vi "Read_Parameters_From_Data_Packet.vi"(8 "error in (no error)":errorcluster, 11 "Data_Packet in":T1={"Packet"={"Raw Bytes"=[], "Checksum"=FALSE, "Direction"=enum."Transmit", "Processed Bytes"=[], "Node ID"=0, "Packet type"=enum."Connection Management", "Frame Data"=0, "Priority"=enum."LOW", "Frame ID"=0}, "Parameters"=[], "Last Received Time (ms)"=0, "Receive count"=0, "Transmit count"=0, "Transmit interval (ms)"=0, "Last Transmitted Time (ms)"=0, "Receive interval (ms)"=0, "Transmit_Mode"=enum."Disabled", "Transmit Enable"=FALSE, "Cyclic Transmit interval (ms)"=0}) -> (0 "error out":errorcluster, 2 "Data Packets Out":T1[](array[typedef]), 3 "Data_Packet out":T1={"Packet"={"Raw Bytes"=[], "Checksum"=FALSE, "Direction"=enum."Transmit", "Processed Bytes"=[], "Node ID"=0, "Packet type"=enum."Connection Management", "Frame Data"=0, "Priority"=enum."LOW", "Frame ID"=0}, "Parameters"=[], "Last Received Time (ms)"=0, "Receive count"=0, "Transmit count"=0, "Transmit interval (ms)"=0, "Last Transmitted Time (ms)"=0, "Receive interval (ms)"=0, "Transmit_Mode"=enum."Disabled", "Transmit Enable"=FALSE, "Cyclic Transmit interval (ms)"=0})   [LabVIEW 2017]
uses:
  Controls/Data Packets/Data_Packet.ctl
  Controls/Packet/Packet.ctl
  Controls/Packet/Packet_Direction.ctl
  Controls/Packet/Packet_Type.ctl
  Controls/Packet/Packet_Priority.ctl
  Controls/Data Packets/Parameter.ctl
  Controls/Data Packets/Parameter_Data_Type.ctl
  Controls/Data Packets/Data_Packet_Transmit_Mode.ctl
  Controls/Data Packets/Data_Packet_FGV_Commands.ctl
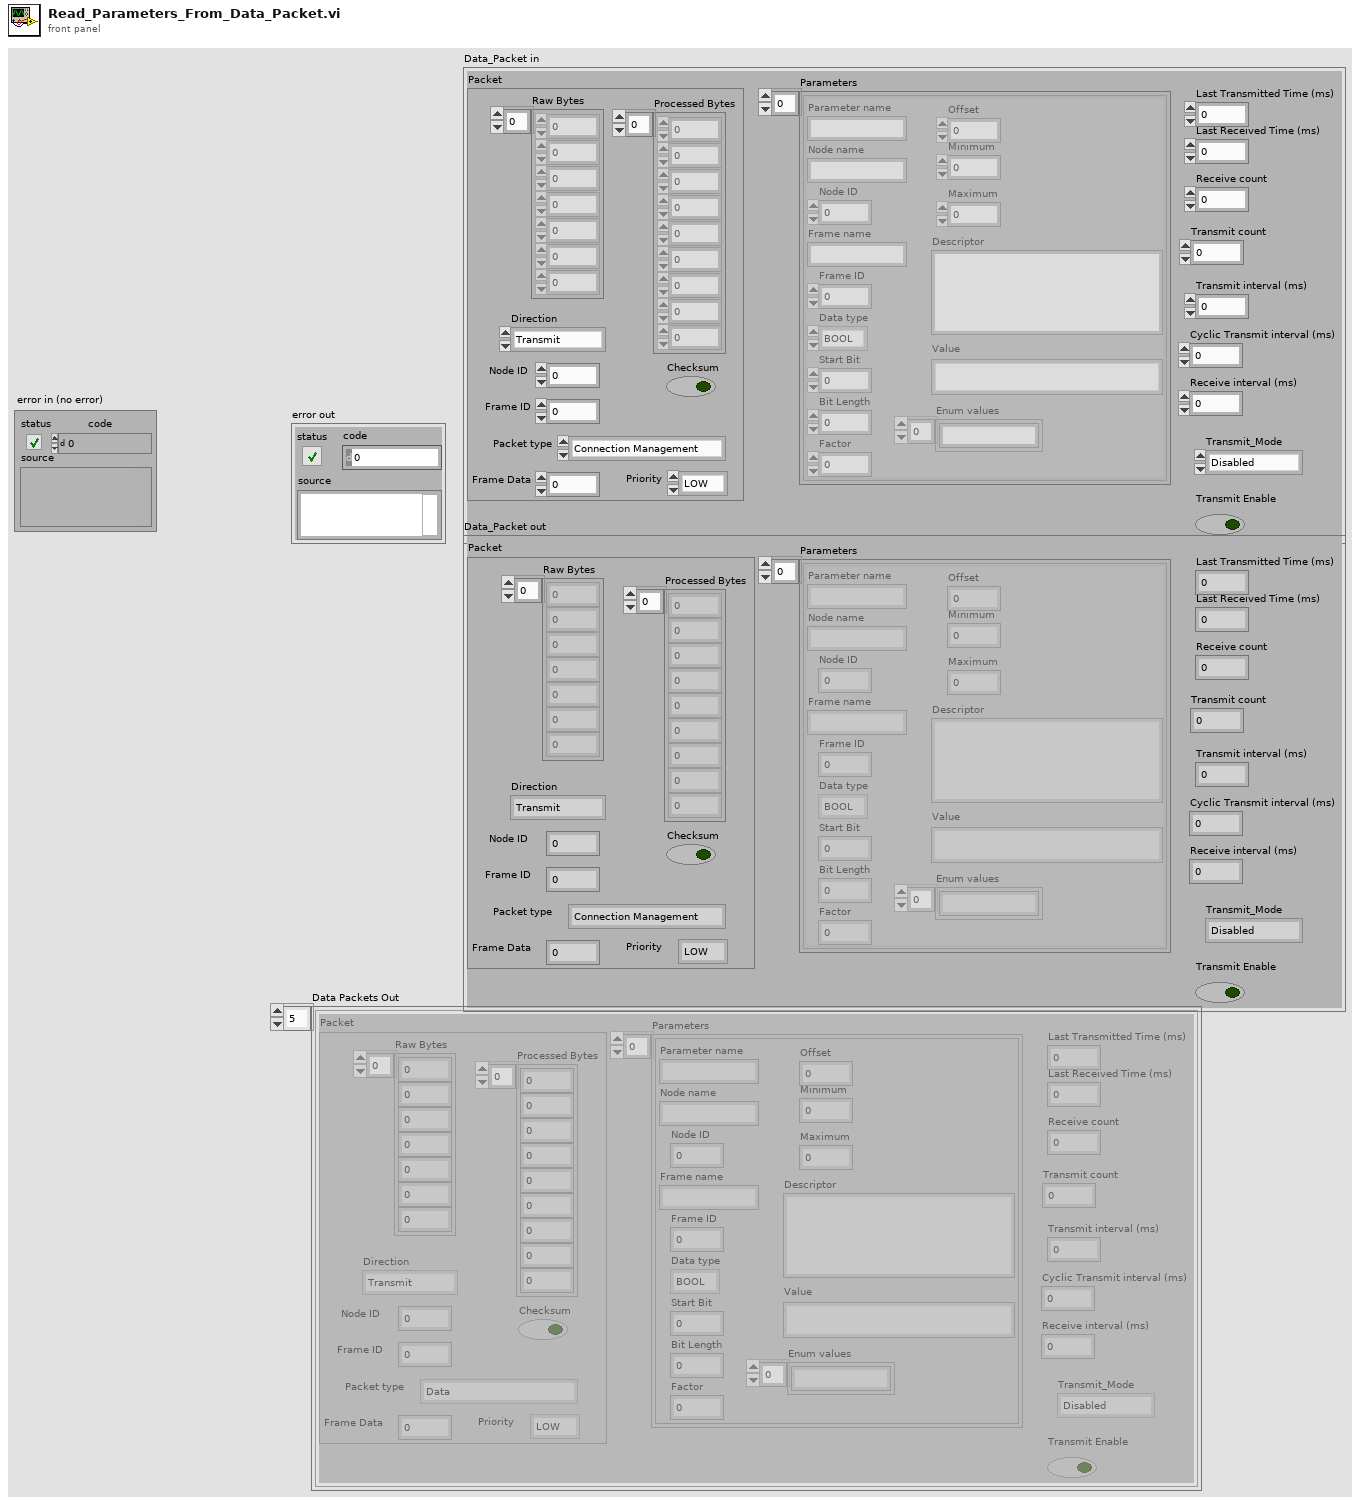
[diagram p1: front panel]
types:
  T1 = typedef "Data_Packet.ctl" = cluster{"Packet":T2, "Parameters":T6[], "Last Received Time (ms)":u64, "Receive count":i32, "Transmit count":i32, "Transmit interval (ms)":u32, "Last Transmitted Time (ms)":u64, "Receive interval (ms)":u32, "Transmit_Mode":T8, "Transmit Enable":bool, "Cyclic Transmit interval (ms)":u32}
  T2 = typedef "Packet.ctl" = cluster{"Raw Bytes":u8[], "Checksum":bool, "Direction":T3, "Processed Bytes":u8[], "Node ID":u8, "Packet type":T4, "Frame Data":u32, "Priority":T5, "Frame ID":u8}
  T3 = typedef "Packet_Direction.ctl" = enum16{"Transmit", "Receive", "Bidirectional"}
  T4 = typedef "Packet_Type.ctl" = enum16{"Data", "Connection Management", "Remote Request", "Error/Status"}
  T5 = typedef "Packet_Priority.ctl" = enum16{"LOW", "HIGH"}
  T6 = typedef "Parameter.ctl" = cluster{"Parameter name":string, "Node name":string, "Node ID":u8, "Frame name":string, "Frame ID":u8, "Data type":T7, "Start Bit":i32, "Bit Length":i32, "Factor":dbl, "Offset":dbl, "Minimum":dbl, "Maximum":dbl, "Descriptor":string, "Enum values":string[], "Value":string}
  T7 = typedef "Parameter_Data_Type.ctl" = enum16{"BOOL", "UNSIGNED", "SIGNED", "FLOAT32", "ENUM"}
  T8 = typedef "Data_Packet_Transmit_Mode.ctl" = enum16{"Disabled", "Single", "Cyclic"}
  T9 = typedef "Data_Packet_FGV_Commands.ctl" = enum16{"Update all parameters from data packets", "Update Packet", "Load", "Read Packet Parameters", "Write Packet Parameters", "Read Packet Parameter", "Write Packet Parameter", "Read Data Packets", "Read Data Packet", "Read Data Packet by Parameter Name", "Get Parameter Node and Frame ID", "Read Data Packet from Node ID and Frame ID"}
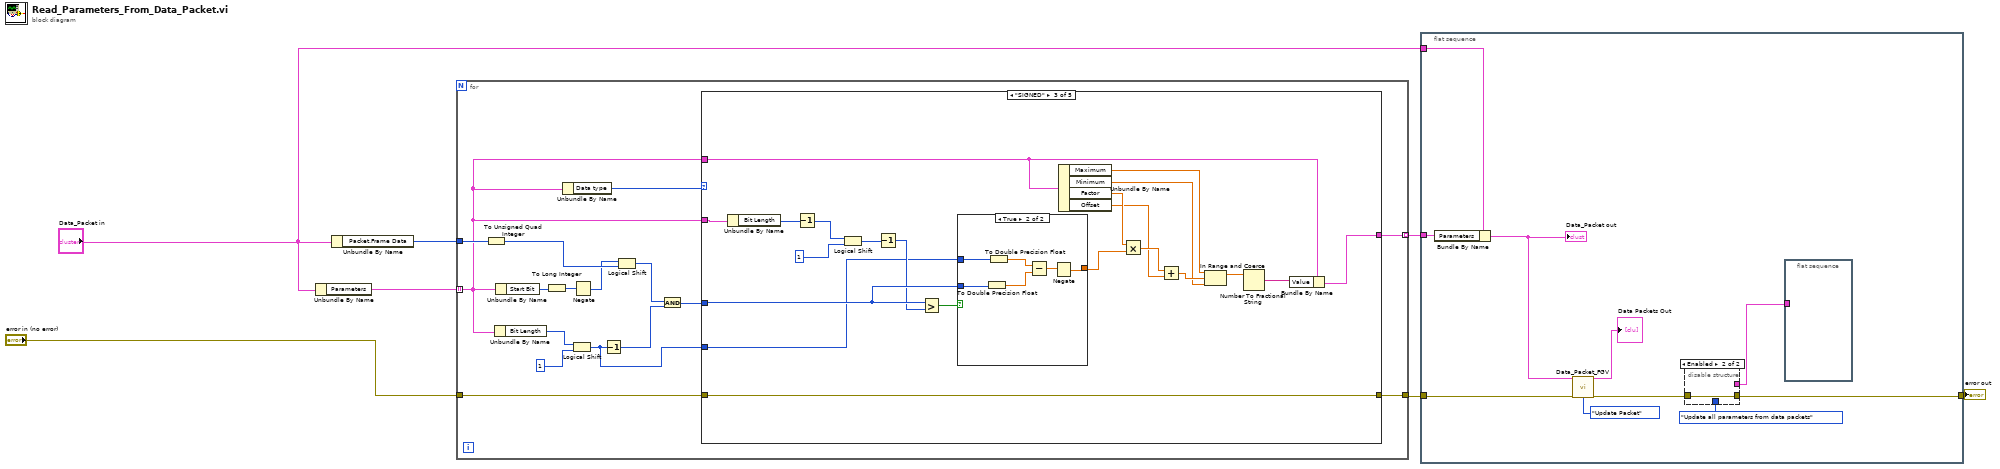
[diagram p0: block diagram]
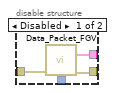
[diagram p2: hidden frame]
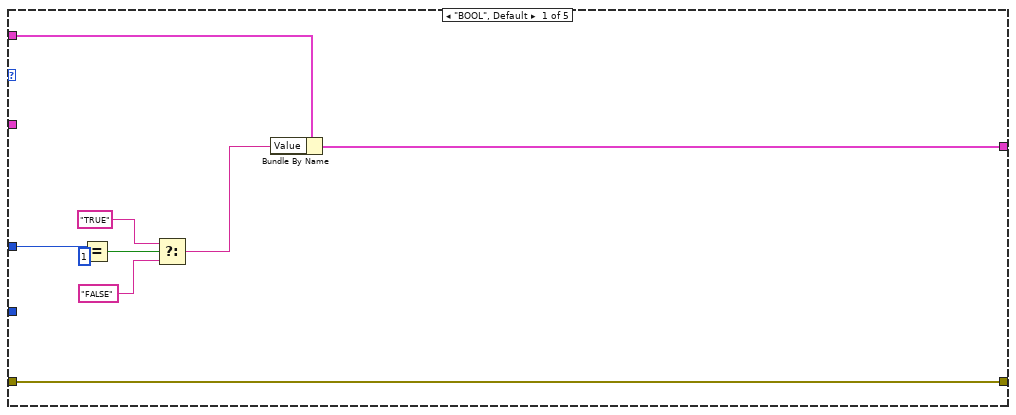
[diagram p3: hidden frame]
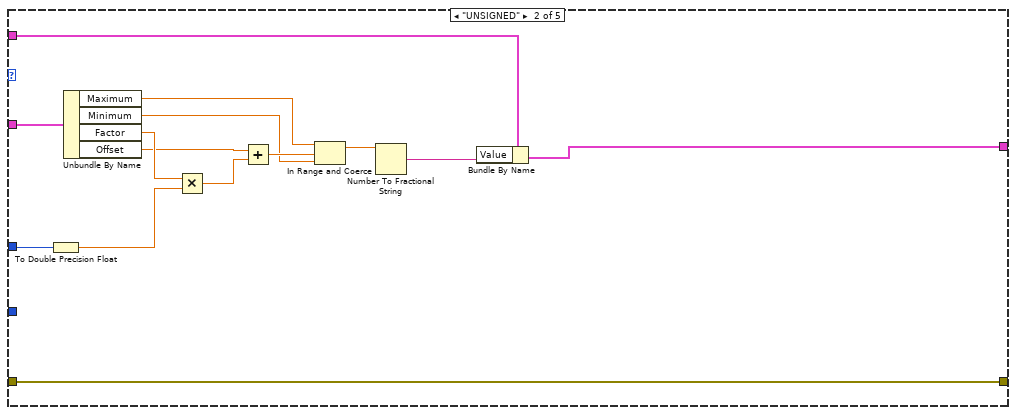
[diagram p4: hidden frame]
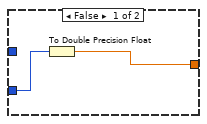
[diagram p5: hidden frame]
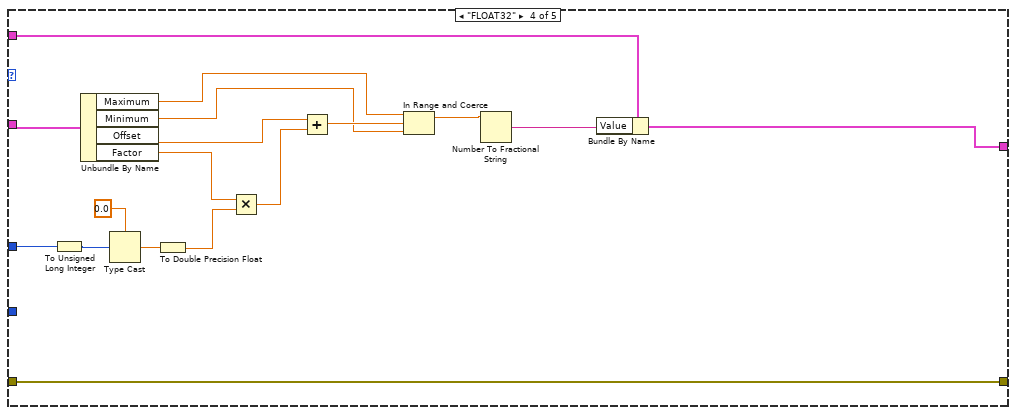
[diagram p6: hidden frame]
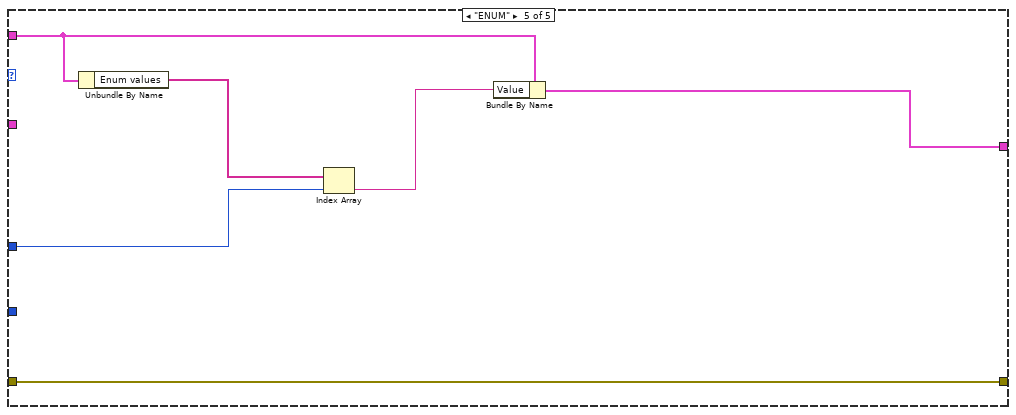
[diagram p7: hidden frame]
diagram:
  n1 = Unbundle By Name("Data_Packet in") -> ("Parameters"=w6:T6[])
  n2 = Unbundle By Name("Data_Packet in") -> ("Packet.Frame Data"=w7:u32)
  n3 = for {
    tunnel: w7 -> [w23]
    tunnel: "error in (no error)" -> [w12]
    tunnel: w6 -> [w10] mode=indexing
    tunnel: [w13] -> w4 mode=indexing
    tunnel: [w11] -> w5
    n4 = To Unsigned Quad Integer(1:w23) -> (0:w22:u64)
    n5 = Unbundle By Name(w10) -> ("Bit Length"=w17:i32)
    n6 = Unbundle By Name(w10) -> ("Start Bit"=w21:i32)
    n7 = To Long Integer(number=w21) -> (32bit integer=w20:i32)
    n8 = Unbundle By Name(w10) -> ("Data type"=w15:T7)
    n9 = Logical Shift(y=w17, x=u64 1) -> (x << y=w8:u64)
    n10 = Negate(x=w20) -> (-x=w19:i32)
    n11 = Decrement(x=w8) -> (x-1=w9:u64)
    n12 = Logical Shift(y=w19, x=w22) -> (x << y=w18:u64)
    n13 = And(x=w18, y=w9) -> (x .and. y?=w14:u64)
    n14 = case shown="\"SIGNED\"" w15 {
      tunnel: w10 -> [w27 w37 w54 w79 w96]
      tunnel: w14 -> [w32 w46 w62 w92 w97]
      tunnel: [w25 w34 w52 w77 w94] -> w13
      tunnel: w12 -> [w24 w33 w56 w76 w93]
      tunnel: [w24 w33 w56 w76 w93] -> w11
      tunnel: w10 -> [_ w45 w67 w87 _]
      tunnel: w8 -> [_ _ w47 _ _]
      frame "BOOL", Default {
        n15 = Equal?(x=w32, y=u64 1) -> (x = y?=w30:bool)
        n16 = Select(t="TRUE", s=w30, f="FALSE") -> (s? t:f=w26:string)
        n17 = Bundle By Name(cluster=w27, "Value"=w26) -> (w25:T6)
      }
      frame "UNSIGNED" {
        n18 = To Double Precision Float(number=w46) -> (double precision float=w43:dbl)
        n19 = Unbundle By Name(w45) -> ("Maximum"=w39:dbl, "Minimum"=w38:dbl, "Factor"=w44:dbl, "Offset"=w42:dbl)
        n20 = Multiply(x=w44, y=w43) -> (x*y=w41:dbl)
        n21 = Add(x=w42, y=w41) -> (x+y=w40:dbl)
        n22 = In Range and Coerce(upper limit=w39, x=w40, lower limit=w38) -> (coerced(x)=w36:dbl)  [unwired: 1 out]
        n23 = Number To Fractional String(number=w36) -> (F-format string=w35:string)  [unwired: 3 in]
        n24 = Bundle By Name(cluster=w37, "Value"=w35) -> (w34:T6)
      }
      frame "SIGNED" {
        n25 = Unbundle By Name(w67) -> ("Bit Length"=w66:i32)
        n26 = Decrement(x=w66) -> (x-1=w65:i32)
        n27 = Logical Shift(y=w65, x=u64 1) -> (x << y=w63:u64)
        n28 = Decrement(x=w63) -> (x-1=w61:u64)
        n29 = Greater?(x=w62, y=w61) -> (0:w55:bool)
        n30 = case shown="True" w55 {
          tunnel: w62 -> [w68 w75]
          tunnel: [w69 w70] -> w59
          tunnel: w47 -> [_ w72]
          frame False {
            n31 = To Double Precision Float(number=w68) -> (double precision float=w69:dbl)
          }
          frame True {
            n32 = To Double Precision Float(number=w75) -> (double precision float=w73:dbl)
            n33 = To Double Precision Float(number=w72) -> (double precision float=w74:dbl)
            n34 = Subtract(x=w74, y=w73) -> (x-y=w71:dbl)
            n35 = Negate(x=w71) -> (-x=w70:dbl)
          }
        }
        n36 = Unbundle By Name(w54) -> ("Maximum"=w49:dbl, "Minimum"=w48:dbl, "Factor"=w60:dbl, "Offset"=w57:dbl)
        n37 = Multiply(x=w60, y=w59) -> (x*y=w58:dbl)
        n38 = Add(x=w58, y=w57) -> (x+y=w50:dbl)
        n39 = In Range and Coerce(upper limit=w49, x=w50, lower limit=w48) -> (coerced(x)=w51:dbl)  [unwired: 1 out]
        n40 = Number To Fractional String(number=w51) -> (F-format string=w53:string)  [unwired: 3 in]
        n41 = Bundle By Name(cluster=w54, "Value"=w53) -> (w52:T6)
      }
      frame "FLOAT32" {
        n42 = To Unsigned Long Integer(number=w92) -> (unsigned 32bit integer=w91:u32)
        n43 = Unbundle By Name(w87) -> ("Maximum"=w82:dbl, "Minimum"=w81:dbl, "Offset"=w85:dbl, "Factor"=w86:dbl)
        n44 = Type Cast(type=sgl 0.0 ("single precision float"), x=w91) -> (*(type *) &x=w89:sgl)
        n45 = To Double Precision Float(number=w89) -> (double precision float=w88:dbl)
        n46 = Multiply(x=w86, y=w88) -> (x*y=w84:dbl)
        n47 = Add(x=w85, y=w84) -> (x+y=w83:dbl)
        n48 = In Range and Coerce(upper limit=w82, x=w83, lower limit=w81) -> (coerced(x)=w80:dbl)  [unwired: 1 out]
        n49 = Number To Fractional String(number=w80) -> (F-format string=w78:string)  [unwired: 3 in]
        n50 = Bundle By Name(cluster=w79, "Value"=w78) -> (w77:T6)
      }
      frame "ENUM" {
        n51 = Unbundle By Name(w96) -> ("Enum values"=w98:string[])
        n52 = Index Array(array=w98, index=w97) -> (element=w95:string)
        n53 = Bundle By Name(cluster=w96, "Value"=w95) -> (w94:T6)
      }
    }
  }
  n54 = flat-sequence {
    tunnel: w5 -> [w108]
    tunnel: w4 -> [w106]
    tunnel: [w101] -> w3
    tunnel: "Data_Packet in" -> [w105]
    frame #0 {
      n55 = Bundle By Name(cluster=w105, "Parameters"=w106) -> (w104:T1)
      "Data_Packet out" <- w104
      n56 = call "Data_Packet_FGV.vi"("Data_Packet In"=w104, "error in (no error)"=w108, "Commands"=Data_Packet_FGV_Commands."Update Packet") -> ("Data Packets Out"=→"Data Packets Out":T1[], "error out"=w103:errorcluster)  [unwired: 7 in, 4 out]
      n57 = disable-structure shown="Enabled" {
        disable-tunnel: w103 -> [w112 w113]
        disable-tunnel: Data_Packet_FGV_Commands."Update all parameters from data packets" ("Commands") -> [w111 _]
        disable-tunnel: [w110 w113] -> w101
        disable-tunnel: [w109 _] -> w100
        frame Disabled {
          n58 = call "Data_Packet_FGV.vi"("error in (no error)"=w112, "Commands"=w111) -> ("Parameters out"=w109:T6[], "error out"=w110:errorcluster)  [unwired: 8 in, 4 out]
        }
        frame Enabled {
        }
      }
      n59 = flat-sequence {
        tunnel: w100 -> [_]
        frame #0 {
        }
      }
    }
  }
  "error out" <- w3
